vi "detect edge.vi"(8 "error in (no error)":errorcluster, 11 "LineCCD in":refnum<class "LineCCD.lvclass">) -> (0 "error out":errorcluster, 2 "fine?":bool, 3 "LineCCD out":refnum<class "LineCCD.lvclass">)   [LabVIEW 2012, in "LineCCD.lvclass"]
uses:
  LineCCD.lvclass
  <vilib>/Analysis/6fits.llb/Curve Fitting Criteria.ctl
  LineCCD.lvclass/LineCCD.ctl
  <vilib>/Analysis/NI_AALPro.lvlib
panel:
  out "fit 2":dbl[](graph)
  out "signal 2":dbl[](graph)
  out "derivata 2":dbl[](graph)
  out "error":i32
  out "fit 1":dbl[](graph)
  out "signal 1":dbl[](graph)
  out "derivata 1":dbl[](graph)
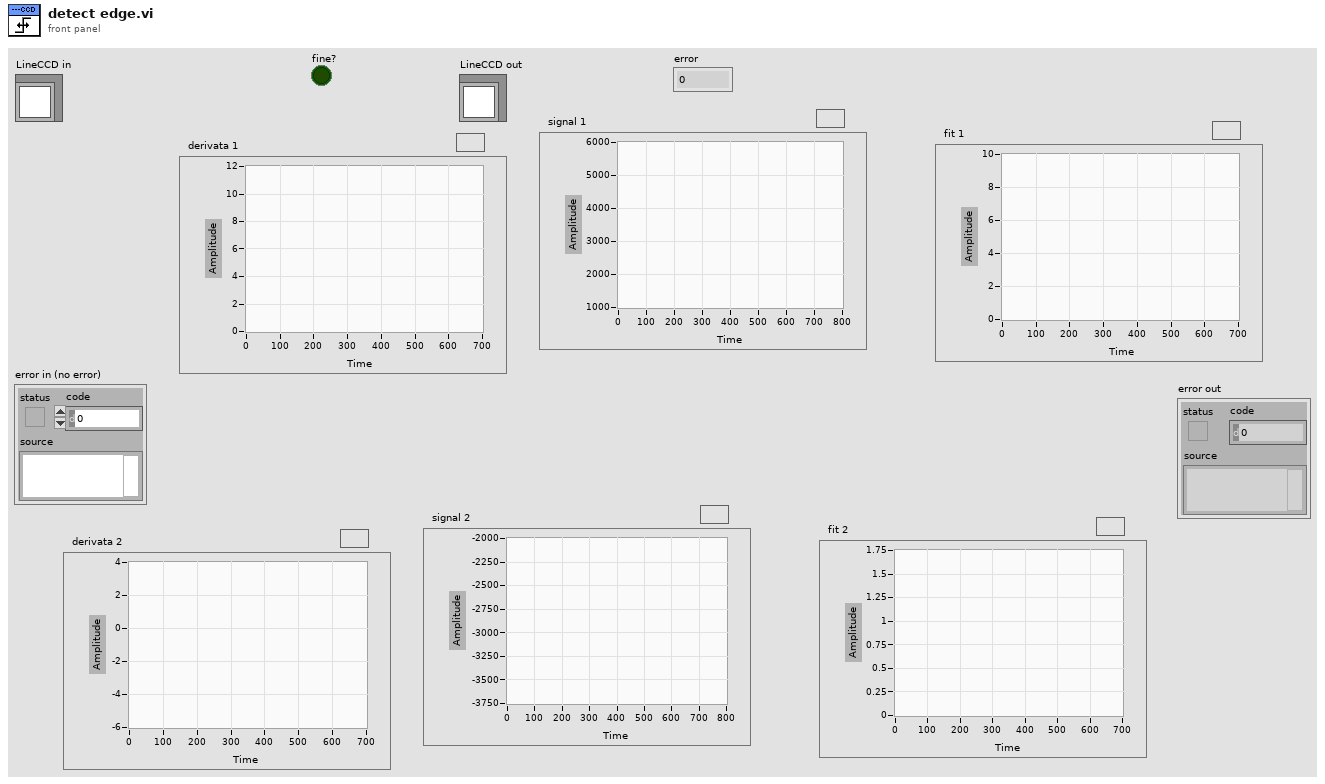
[diagram p1: front panel]
types:
  T1 = cluster{"initial amplitude":dbl, "initial center":dbl, "initial standard deviation":dbl, "offset":dbl}
  T2 = typedef "NI_AALPro.lvlib/Curve Fitting Criteria.ctl" = u16
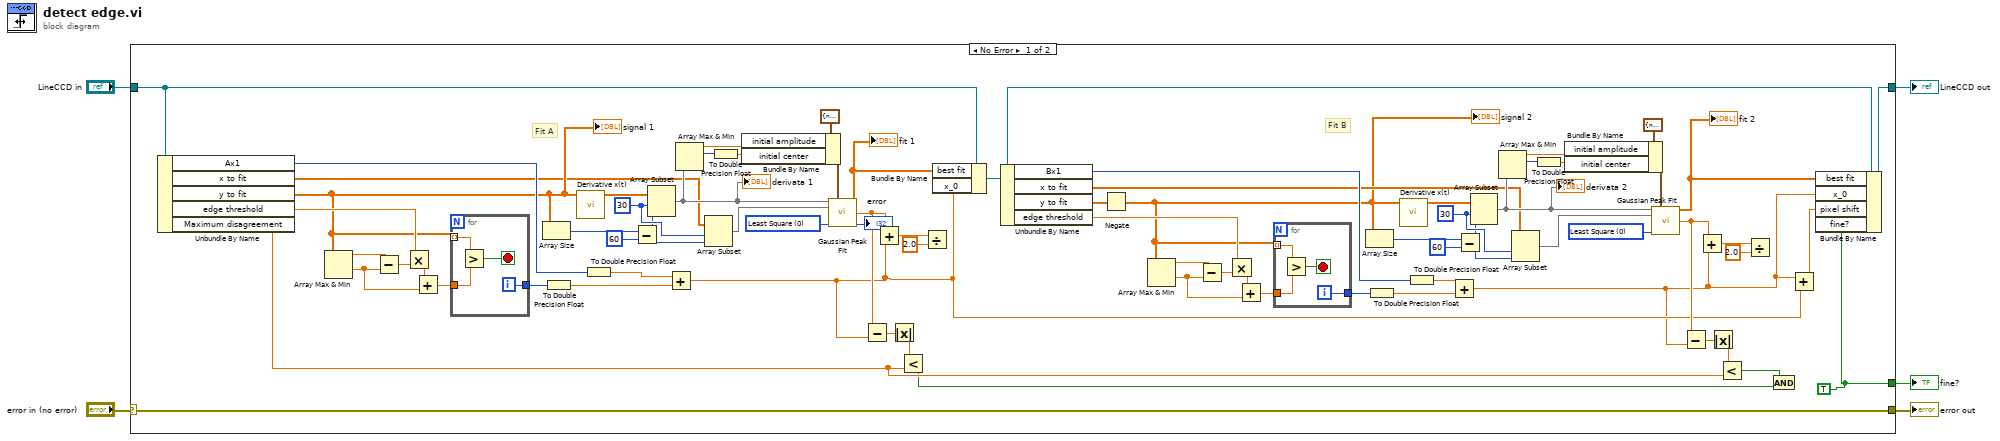
[diagram p0: block diagram]
diagram:
  n1 = case shown="No Error" "error in (no error)" {
    selector: "error in (no error)" -> [w80 w90]
    tunnel: [w80 w90] -> w4
    tunnel: [w41 w89] -> w2
    tunnel: "LineCCD in" -> [w62 w89]
    tunnel: [w10 _] -> w1
    frame No Error {
      w10 = TRUE
      w47 = T2 0 items=["Least Square", "Least Absolute Residual", "Bisquare"] ("method")
      w22 = 30 ("index")
      w67 = T2 0 items=["Least Square", "Least Absolute Residual", "Bisquare"] ("method")
      w29 = 30 ("index")
      # "Fit A"
      # "Fit B"
      n2 = Unbundle By Name(w62) -> ("Ax1"=w64:i32, "x to fit"=w27:dbl[], "y to fit"=w32:dbl[], "edge threshold"=w77:dbl, "Maximum disagreement"=w36:dbl)
      "signal 1" <- w32
      n3 = Array Max & Min(array=w32) -> (max value=w79:dbl, min value=w75:dbl)  [unwired: 2 out]
      n4 = Subtract(x=w79, y=w75) -> (x-y=w78:dbl)
      n5 = Multiply(x=w77, y=w78) -> (x*y=w76:dbl)
      n6 = Add(x=w76, y=w75) -> (x+y=w74:dbl)
      n7 = for {
        tunnel: w32 -> [w88] mode=indexing
        tunnel: w74 -> [w87]
        tunnel: [w85] -> w66
        i -> [w85]
        stop <- w86 stop-if-true
        n8 = Greater?(x=w88, y=w87) -> (0:w86:bool)
      }
      n9 = Array Size(array=w32) -> (size(s)=w73:i32)
      n10 = To Double Precision Float(number=w66) -> (double precision float=w18:dbl)
      n11 = call <vilib>:"Derivative x(t).vi"("X"=w32) -> ("dX/dt"=w31:dbl[])  [unwired: 9 in, 1 out]
      n12 = To Double Precision Float(number=w64) -> (double precision float=w19:dbl)
      n13 = Subtract(x=w73, y=60) -> (x-y=w28:i32)
      n14 = Array Subset(array=w31, index=w29, length=w28) -> (w33:dbl[])
      "derivata 1" <- w33
      n15 = Add(x=w19, y=w18) -> (x+y=w7:dbl)
      n16 = Array Max & Min(array=w33) -> (max value=w70:dbl, max index (indices)=w68:i32)  [unwired: 2 out]
      n17 = Array Subset(array=w27, index=w29, length=w28) -> (w26:dbl[])
      n18 = To Double Precision Float(number=w68) -> (double precision float=w69:dbl)
      n19 = Bundle By Name(cluster=T1 {"initial amplitude"=nan, "initial center"=nan, "initial standard deviation"=nan, "offset"=nan} ("initial guess"), "initial amplitude"=w70, "initial center"=w69) -> (w71:T1)
      n20 = call <vilib>:"Gaussian Peak Fit.vi"("Y"=w33, "initial guess"=w71, "X"=w26, "method"=w67) -> ("Best Gaussian Fit"=w24:dbl[], "center"=w8:dbl, "error"=→"error":i32)  [unwired: 5 in, 4 out]
      "fit 1" <- w24
      n21 = Subtract(x=w8, y=w7) -> (x-y=w40:dbl)
      n22 = Add(x=w7, y=w8) -> (x+y=w65:dbl)
      n23 = Absolute Value(x=w40) -> (abs(x)=w39:dbl)
      n24 = Less?(x=w39, y=w36) -> (x < y?=w34:bool)
      n25 = Divide(x=w65, y=2.0) -> ()  [unwired: 1 out]
      n26 = Bundle By Name(cluster=w62, "best fit"=w24, "x_0"=w7) -> (w42:refnum<class "LineCCD.lvclass">)
      n27 = Unbundle By Name(w42) -> ("Bx1"=w44:i32, "x to fit"=w13:dbl[], "y to fit"=w55:dbl[], "edge threshold"=w59:dbl)
      n28 = Negate(x=w55) -> (-x=w12:dbl[])
      "signal 2" <- w12
      n29 = Array Max & Min(array=w12) -> (max value=w61:dbl, min value=w57:dbl)  [unwired: 2 out]
      n30 = Subtract(x=w61, y=w57) -> (x-y=w60:dbl)
      n31 = Multiply(x=w59, y=w60) -> (x*y=w58:dbl)
      n32 = Add(x=w58, y=w57) -> (x+y=w56:dbl)
      n33 = for {
        tunnel: w12 -> [w84] mode=indexing
        tunnel: w56 -> [w83]
        tunnel: [w81] -> w46
        i -> [w81]
        stop <- w82 stop-if-true
        n34 = Greater?(x=w84, y=w83) -> (0:w82:bool)
      }
      n35 = Array Size(array=w12) -> (size(s)=w53:i32)
      n36 = To Double Precision Float(number=w46) -> (double precision float=w16:dbl)
      n37 = call <vilib>:"Derivative x(t).vi"("X"=w12) -> ("dX/dt"=w54:dbl[])  [unwired: 9 in, 1 out]
      n38 = To Double Precision Float(number=w44) -> (double precision float=w17:dbl)
      n39 = Add(x=w17, y=w16) -> (x+y=w6:dbl)
      n40 = Subtract(x=w53, y=60) -> (x-y=w20:i32)
      n41 = Array Subset(array=w54, index=w22, length=w20) -> (w14:dbl[])
      "derivata 2" <- w14
      n42 = Array Max & Min(array=w14) -> (max value=w50:dbl, max index (indices)=w48:i32)  [unwired: 2 out]
      n43 = Array Subset(array=w13, index=w22, length=w20) -> (w23:dbl[])
      n44 = To Double Precision Float(number=w48) -> (double precision float=w49:dbl)
      n45 = Bundle By Name(cluster=T1 {"initial amplitude"=nan, "initial center"=nan, "initial standard deviation"=nan, "offset"=nan} ("initial guess"), "initial amplitude"=w50, "initial center"=w49) -> (w51:T1)
      n46 = call <vilib>:"Gaussian Peak Fit.vi"("Y"=w14, "initial guess"=w51, "X"=w23, "method"=w47) -> ("Best Gaussian Fit"=w15:dbl[], "center"=w9:dbl)  [unwired: 5 in, 5 out]
      "fit 2" <- w15
      n47 = Subtract(x=w9, y=w6) -> (x-y=w38:dbl)
      n48 = Add(x=w6, y=w9) -> (x+y=w45:dbl)
      n49 = Absolute Value(x=w38) -> (abs(x)=w37:dbl)
      n50 = Less?(x=w37, y=w36) -> (x < y?=w35:bool)
      n51 = Divide(x=w45, y=2.0) -> ()  [unwired: 1 out]
      n52 = And(x=w35, y=w34) -> ()  [unwired: 1 out]
      n53 = Add(x=w6, y=w7) -> (x+y=w11:dbl)
      n54 = Bundle By Name(cluster=w42, "best fit"=w15, "x_0"=w6, "pixel shift"=w11, "fine?"=w10) -> (w41:refnum<class "LineCCD.lvclass">)
    }
    frame Error {
    }
  }
  "error out" <- w4
  "LineCCD out" <- w2
  "fine?" <- w1
